vi "Main.vi"() -> ()   [LabVIEW 2017]
uses:
  <userlib>/dynamixel/dynamixel.lvlib
panel:
  in  "GO":bool
  out "Temp 2":cluster{"pos1":dbl, "pos2":dbl, "pos3":dbl}
  out "Temp":cluster{"pos1":dbl, "pos2":dbl, "pos3":dbl}
  in  "A <--> B":bool
  out "POS":cluster{"X":dbl, "Y":dbl, "Z":dbl}
  in  "Home":bool
  in  "P -> B":bool
  in  "P -> A":bool
  in  "P":cluster{"Px":dbl, "Py":dbl, "Pz":dbl}={"Px"=0.0, "Py"=0.0, "Pz"=287.0} {"Pz" format="%#.3f"; "Py" format="%#.3f"; "Px" format="%#.3f"}
  in  "A":cluster{"Bx":dbl, "By":dbl, "Bz":dbl} {"Bz" format="%#.3f"; "By" format="%#.3f"; "Bx" format="%#.3f"}
  in  "B":cluster{"Ax":dbl, "Ay":dbl, "Az":dbl} {"Az" format="%#.3f"; "Ay" format="%#.3f"; "Ax" format="%#.3f"}
  in  "Pt to Pt (GO)":bool
  in  "# of points(A to B)":i16=11
  in  "theta1a":dbl min=-150.0 max=150.0 format="%#.3f"
  in  "theta2a":dbl min=-150.0 max=150.0 format="%#.3f"
  in  "theta3a":dbl min=-150.0 max=150.0 format="%#.3f"
  in  "theta4a":dbl(knob) min=-140.0 max=140.0 scale=120.0..-120.0
  in  "devIndex":i32=46
  in  "STOP":bool
  in  "Mode Control":u16(ring) items=["Joint Space", "Cartesian Space", "Point to Point(Joint Space)", "Point to Point(Cartesian Space)", "Duplicate Position", "Home"]
  in  "constant":cluster{"d1":dbl, "a2":dbl, "a3":dbl}={"d1"=100.0, "a2"=67.0, "a3"=120.0}
  in  "ID":i16[](array[numeric])=[1, 2, 3, 4]
  # "¾÷±ñ¤âÁu±±¨îHMI"
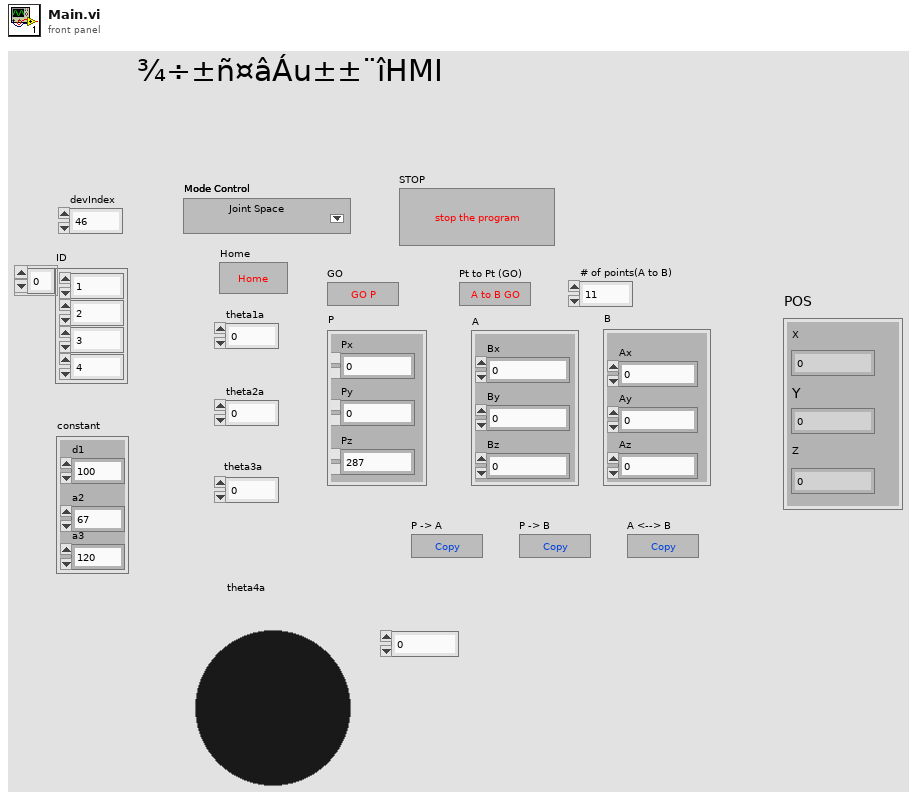
[diagram p1: front panel]
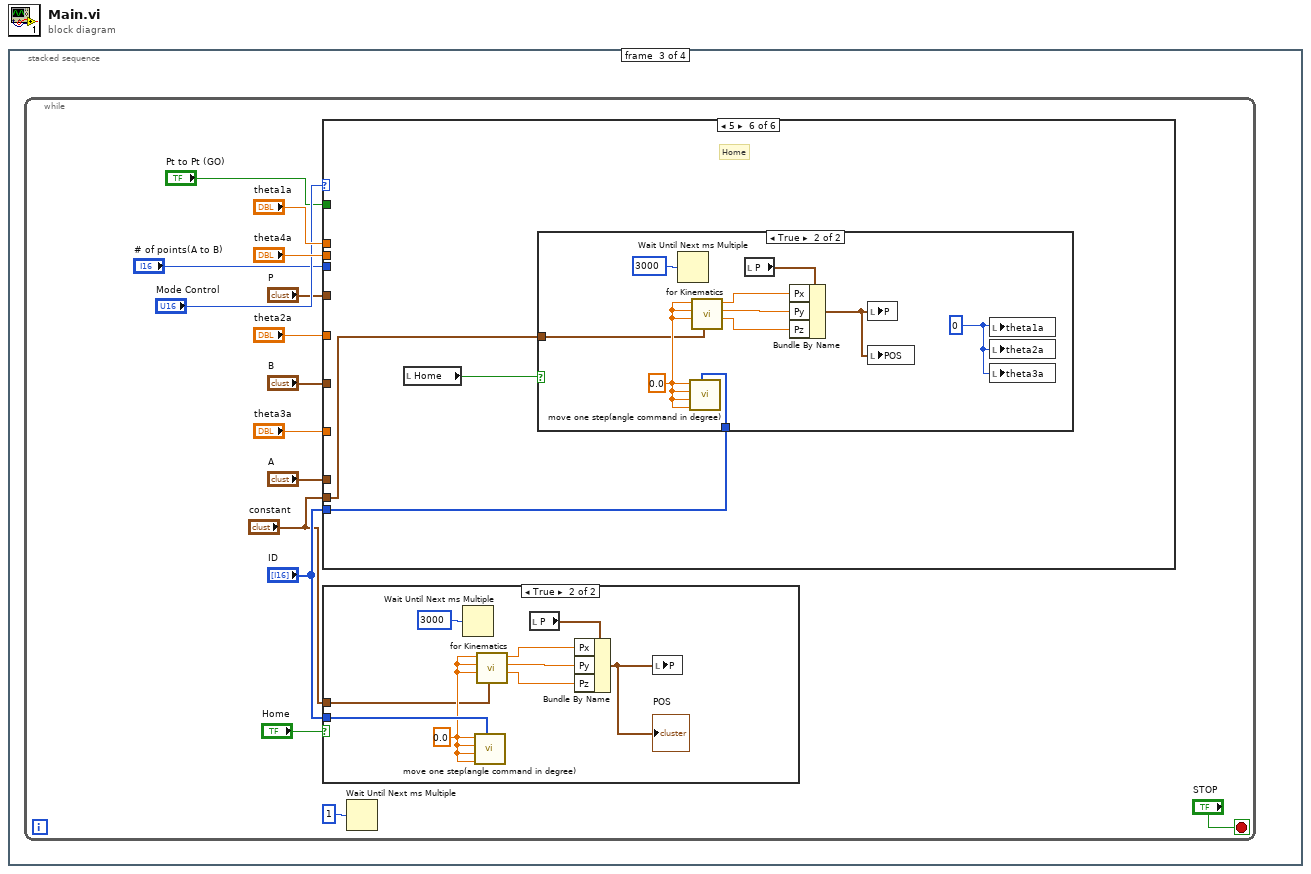
[diagram p0: block diagram]
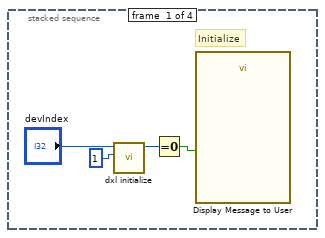
[diagram p2: hidden frame]
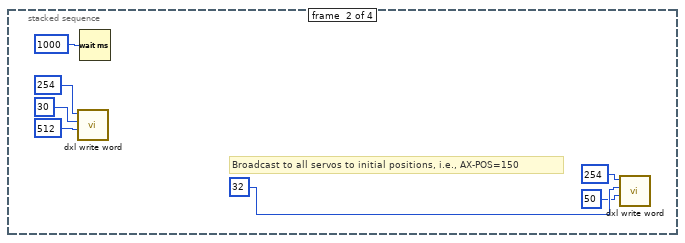
[diagram p3: hidden frame]
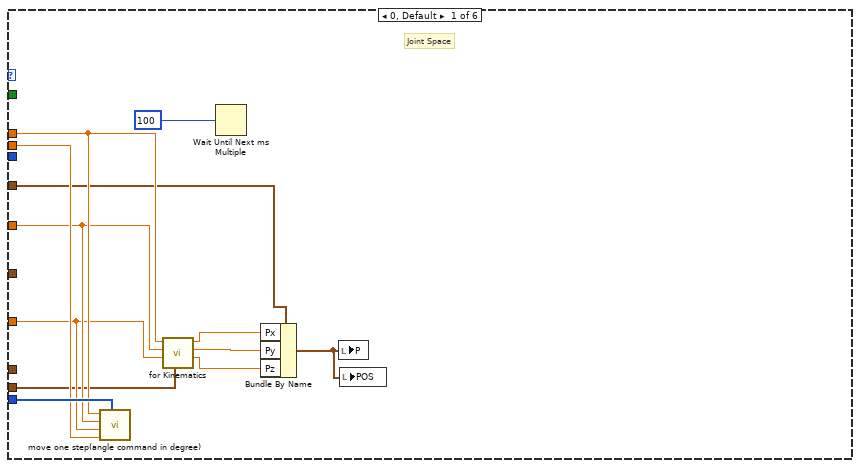
[diagram p5: hidden frame]
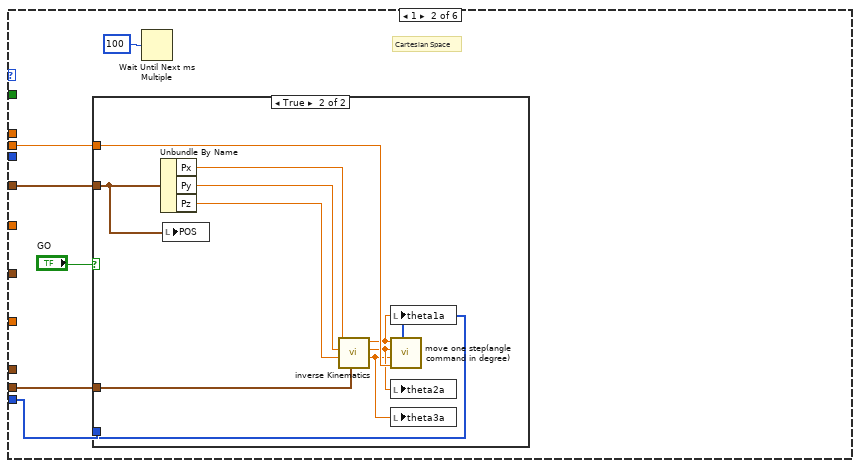
[diagram p6: hidden frame]
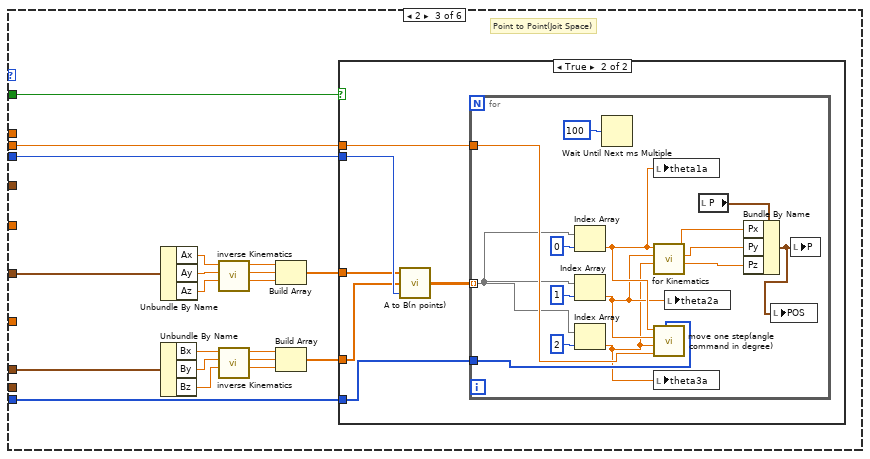
[diagram p8: hidden frame]
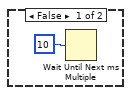
[diagram p9: hidden frame]
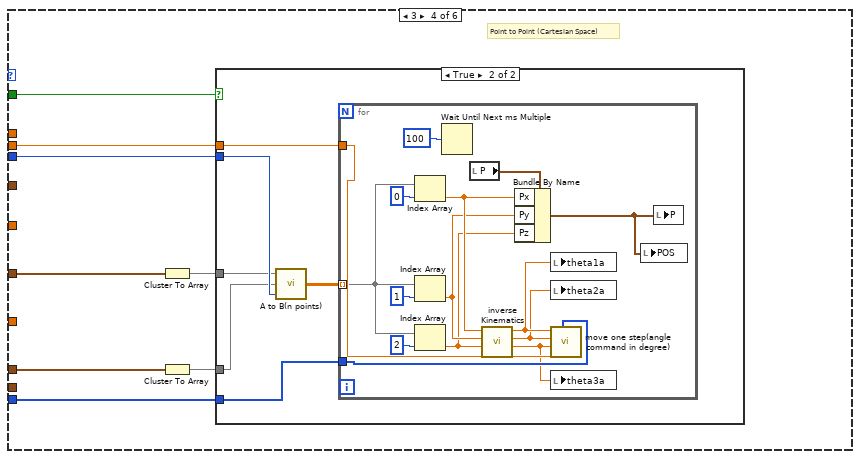
[diagram p10: hidden frame]
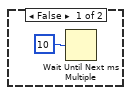
[diagram p11: hidden frame]
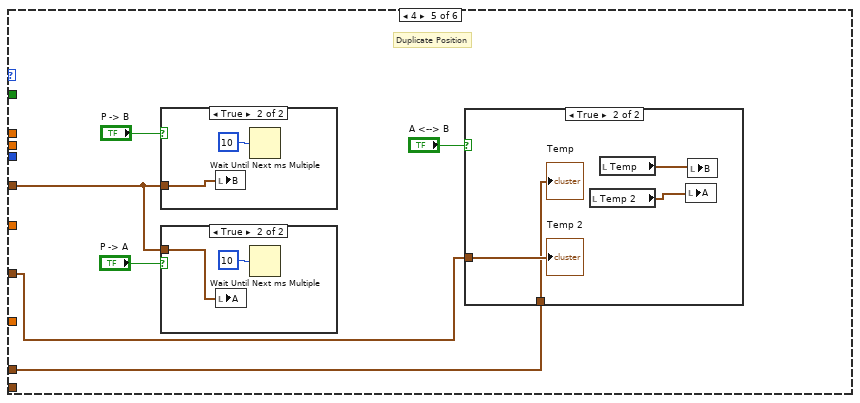
[diagram p12: hidden frame]
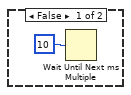
[diagram p14: hidden frame]
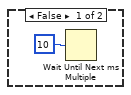
[diagram p15: hidden frame]
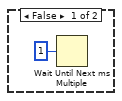
[diagram p16: hidden frame]
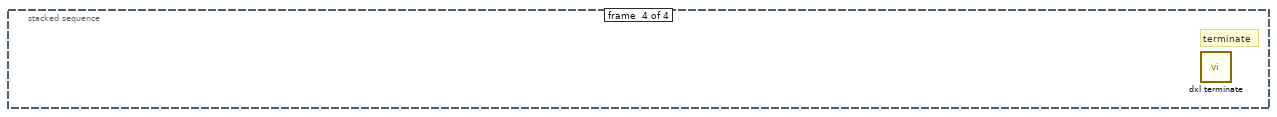
[diagram p17: hidden frame]
diagram:
  n1 = stacked-sequence {
    frame #0 {
      # "Initialize"
      n2 = call <userlib>:"dxl initialize.vi"("baudnum"=1, "devIndex"="devIndex") -> ("function return"=w3:i32)  [unwired: 9 in]
      n3 = Equal To 0?(x=w3) -> (x = 0?=w2:bool)
      n4 = call "Display Message to User"("Enable"=w2) -> ()  [unwired: 9 in, 2 out]
    }
    frame #1 {
      # "Broadcast to all servos to initial positions, i.e., AX-POS=150"
      n5 = call <userlib>:"dxl write word.vi"("value"=512, "address"=30, "id"=254) -> ()  [unwired: 9 in]
      n6 = Wait (ms)(milliseconds to wait=u32 1000) -> ()  [unwired: 1 out]
      n7 = call <userlib>:"dxl write word.vi"("value"=50, "address"=32, "id"=254) -> ()  [unwired: 9 in]
    }
    frame #2 {
      n8 = while {
        stop <- "STOP" stop-if-true
        n9 = case shown="5" "Mode Control" {
          tunnel: "theta1a" -> [w45 _ _ _ _ _]
          tunnel: "theta2a" -> [w44 _ _ _ _ _]
          tunnel: "theta3a" -> [w43 _ _ _ _ _]
          tunnel: "theta4a" -> [w46 w52 w82 w112 _ _]
          tunnel: "ID" -> [w47 w49 w83 w113 _ w153]
          tunnel: "constant" -> [w42 w53 _ _ _ w152]
          tunnel: "# of points(A to B)" -> [_ _ w81 w111 _ _]
          tunnel: "B" -> [_ _ w77 w110 w138 _]
          tunnel: "Pt to Pt (GO)" -> [_ _ w65 w107 _ _]
          tunnel: "P" -> [w37 w50 _ _ w139 _]
          tunnel: "A" -> [_ _ w64 w106 w137 _]
          frame 0, Default {
            # "Joint Space"
            n10 = call "move one step(angle command in degree).vi"("ID"=w47, "theta4a"=w46, "theta3a"=w43, "theta2a"=w44, "theta1a"=w45) -> ()  [unwired: 6 in]
            n11 = call "for Kinematics.vi"("constant"=w42, "theta3a"=w43, "theta2a"=w44, "theta1a"=w45) -> ("Pz"=w39:dbl, "Py"=w40:dbl, "Px"=w41:dbl)  [unwired: 5 in]
            n12 = Wait Until Next ms Multiple(millisecond multiple=u32 100) -> ()  [unwired: 1 out]
            n13 = Bundle By Name(cluster=w37, "Px"=w41, "Py"=w40, "Pz"=w39) -> (w36:cluster{"Px":dbl, "Py":dbl, "Pz":dbl})
            n14 = local write "P"(w36) -> ()
            n15 = local write "POS"(w36) -> ()
          }
          frame 1 {
            # "Cartesian Space"
            n16 = case shown="True" "GO" {
              tunnel: w53 -> [_ w63]
              tunnel: w52 -> [_ w62]
              tunnel: w50 -> [_ w55]
              tunnel: w49 -> [_ w54]
              frame False {
              }
              frame True {
                n17 = Unbundle By Name(w55) -> ("Px"=w58:dbl, "Py"=w57:dbl, "Pz"=w56:dbl)
                n18 = local write "POS"(w55) -> ()
                n19 = call "inverse Kinematics.vi"("constant"=w63, "Pz"=w56, "Py"=w57, "Px"=w58) -> ("theta3a"=w59:dbl, "theta2a"=w60:dbl, "theta1a"=w61:dbl)  [unwired: 5 in]
                n20 = local write "theta1a"(w61) -> ()
                n21 = call "move one step(angle command in degree).vi"("ID"=w54, "theta4a"=w62, "theta3a"=w59, "theta2a"=w60, "theta1a"=w61) -> ()  [unwired: 6 in]
                n22 = local write "theta2a"(w60) -> ()
                n23 = local write "theta3a"(w59) -> ()
              }
            }
            n24 = Wait Until Next ms Multiple(millisecond multiple=u32 100) -> ()  [unwired: 1 out]
          }
          frame 2 {
            # "Point to Point(Joit Space)"
            n25 = Unbundle By Name(w77) -> ("Ax"=w76:dbl, "Ay"=w75:dbl, "Az"=w74:dbl)
            n26 = Unbundle By Name(w64) -> ("Bx"=w80:dbl, "By"=w79:dbl, "Bz"=w78:dbl)
            n27 = call "inverse Kinematics.vi"("Pz"=w74, "Py"=w75, "Px"=w76) -> ("theta3a"=w71:dbl, "theta2a"=w72:dbl, "theta1a"=w73:dbl)  [unwired: 6 in]
            n28 = call "inverse Kinematics.vi"("Pz"=w78, "Py"=w79, "Px"=w80) -> ("theta3a"=w68:dbl, "theta2a"=w69:dbl, "theta1a"=w70:dbl)  [unwired: 6 in]
            n29 = Build Array(w73, w72, w71) -> (w66:dbl[])
            n30 = Build Array(w70, w69, w68) -> (w67:dbl[])
            n31 = case shown="True" w65 {
              tunnel: w83 -> [_ w90]
              tunnel: w82 -> [_ w89]
              tunnel: w81 -> [_ w87]
              tunnel: w67 -> [_ w85]
              tunnel: w66 -> [_ w86]
              frame False {
                n32 = Wait Until Next ms Multiple(millisecond multiple=u32 10) -> ()  [unwired: 1 out]
              }
              frame True {
                n33 = call "A to B(n points).vi"("N"=w87, "B"=w85, "A"=w86) -> ("R"=w88:dbl[][])
                n34 = for {
                  tunnel: w90 -> [w105]
                  tunnel: w89 -> [w103]
                  tunnel: w88 -> [w102] mode=indexing
                  n35 = Index Array(array=w102, index=0) -> (element=w98:dbl)
                  n36 = Index Array(array=w102, index=1) -> (element=w97:dbl)
                  n37 = Index Array(array=w102, index=2) -> (element=w96:dbl)
                  n38 = Wait Until Next ms Multiple(millisecond multiple=u32 100) -> ()  [unwired: 1 out]
                  n39 = local write "theta1a"(w98) -> ()
                  n40 = call "for Kinematics.vi"("theta3a"=w96, "theta2a"=w97, "theta1a"=w98) -> ("Pz"=w93:dbl, "Py"=w94:dbl, "Px"=w95:dbl)  [unwired: 6 in]
                  n41 = call "move one step(angle command in degree).vi"("ID"=w105, "theta4a"=w103, "theta3a"=w96, "theta2a"=w97, "theta1a"=w98) -> ()  [unwired: 6 in]
                  n42 = local write "theta3a"(w96) -> ()
                  n43 = local write "theta2a"(w97) -> ()
                  n44 = local read "P"() -> (w92:cluster{"Px":dbl, "Py":dbl, "Pz":dbl})
                  n45 = Bundle By Name(cluster=w92, "Px"=w95, "Py"=w94, "Pz"=w93) -> (w91:cluster{"Px":dbl, "Py":dbl, "Pz":dbl})
                  n46 = local write "POS"(w91) -> ()
                  n47 = local write "P"(w91) -> ()
                }
              }
            }
          }
          frame 3 {
            # "Point to Point (Cartesian Space)"
            n48 = Cluster To Array(cluster=w110) -> (array=w109:dbl[])
            n49 = Cluster To Array(cluster=w106) -> (array=w108:dbl[])
            n50 = case shown="True" w107 {
              tunnel: w113 -> [_ w120]
              tunnel: w112 -> [_ w119]
              tunnel: w111 -> [_ w117]
              tunnel: w109 -> [_ w116]
              tunnel: w108 -> [_ w115]
              frame False {
                n51 = Wait Until Next ms Multiple(millisecond multiple=u32 10) -> ()  [unwired: 1 out]
              }
              frame True {
                n52 = call "A to B(n points).vi"("N"=w117, "B"=w115, "A"=w116) -> ("R"=w118:dbl[][])
                n53 = for {
                  tunnel: w120 -> [w135]
                  tunnel: w119 -> [w133]
                  tunnel: w118 -> [w132] mode=indexing
                  n54 = Index Array(array=w132, index=0) -> (element=w125:dbl)
                  n55 = Index Array(array=w132, index=1) -> (element=w124:dbl)
                  n56 = Index Array(array=w132, index=2) -> (element=w123:dbl)
                  n57 = Wait Until Next ms Multiple(millisecond multiple=u32 100) -> ()  [unwired: 1 out]
                  n58 = local read "P"() -> (w122:cluster{"Px":dbl, "Py":dbl, "Pz":dbl})
                  n59 = call "inverse Kinematics.vi"("Pz"=w123, "Py"=w124, "Px"=w125) -> ("theta3a"=w126:dbl, "theta2a"=w127:dbl, "theta1a"=w128:dbl)  [unwired: 6 in]
                  n60 = Bundle By Name(cluster=w122, "Px"=w125, "Py"=w124, "Pz"=w123) -> (w121:cluster{"Px":dbl, "Py":dbl, "Pz":dbl})
                  n61 = local write "theta1a"(w128) -> ()
                  n62 = local write "theta2a"(w127) -> ()
                  n63 = call "move one step(angle command in degree).vi"("ID"=w135, "theta4a"=w133, "theta3a"=w126, "theta2a"=w127, "theta1a"=w128) -> ()  [unwired: 6 in]
                  n64 = local write "theta3a"(w126) -> ()
                  n65 = local write "POS"(w121) -> ()
                  n66 = local write "P"(w121) -> ()
                }
              }
            }
          }
          frame 4 {
            # "Duplicate Position"
            n67 = case shown="True" "P -> B" {
              tunnel: w139 -> [_ w147]
              frame False {
                n68 = Wait Until Next ms Multiple(millisecond multiple=u32 10) -> ()  [unwired: 1 out]
              }
              frame True {
                n69 = local write "B"(w147) -> ()
                n70 = Wait Until Next ms Multiple(millisecond multiple=u32 10) -> ()  [unwired: 1 out]
              }
            }
            n71 = case shown="True" "P -> A" {
              tunnel: w139 -> [_ w150]
              frame False {
                n72 = Wait Until Next ms Multiple(millisecond multiple=u32 10) -> ()  [unwired: 1 out]
              }
              frame True {
                n73 = local write "A"(w150) -> ()
                n74 = Wait Until Next ms Multiple(millisecond multiple=u32 10) -> ()  [unwired: 1 out]
              }
            }
            n75 = case shown="True" "A <--> B" {
              tunnel: w138 -> [_ w145]
              tunnel: w137 -> [_ w144]
              frame False {
              }
              frame True {
                n76 = local read "Temp 2"() -> (w142:cluster{"pos1":dbl, "pos2":dbl, "pos3":dbl})
                n77 = local read "Temp"() -> (w143:cluster{"pos1":dbl, "pos2":dbl, "pos3":dbl})
                n78 = local write "A"(w142) -> ()
                n79 = local write "B"(w143) -> ()
                "Temp" <- w144
                "Temp 2" <- w145
              }
            }
          }
          frame 5 {
            # "Home"
            n80 = local read "Home"() -> (w154:bool)
            n81 = case shown="True" w154 {
              tunnel: w153 -> [_ w159]
              tunnel: w152 -> [_ w158]
              frame False {
                n82 = Wait Until Next ms Multiple(millisecond multiple=u32 1) -> ()  [unwired: 1 out]
              }
              frame True {
                w156 = 0
                w165 = 0.0 ("theta1a")
                n83 = Wait Until Next ms Multiple(millisecond multiple=u32 3000) -> ()  [unwired: 1 out]
                n84 = call "move one step(angle command in degree).vi"("ID"=w159, "theta4a"=w165, "theta3a"=w165, "theta2a"=w165, "theta1a"=w165) -> ()  [unwired: 6 in]
                n85 = call "for Kinematics.vi"("constant"=w158, "theta3a"=w165, "theta2a"=w165, "theta1a"=w165) -> ("Pz"=w162:dbl, "Py"=w163:dbl, "Px"=w164:dbl)  [unwired: 5 in]
                n86 = local read "P"() -> (w160:cluster{"Px":dbl, "Py":dbl, "Pz":dbl})
                n87 = Bundle By Name(cluster=w160, "Px"=w164, "Py"=w163, "Pz"=w162) -> (w157:cluster{"Px":dbl, "Py":dbl, "Pz":dbl})
                n88 = local write "P"(w157) -> ()
                n89 = local write "POS"(w157) -> ()
                n90 = local write "theta1a"(w156) -> ()
                n91 = local write "theta2a"(w156) -> ()
                n92 = local write "theta3a"(w156) -> ()
              }
            }
          }
        }
        n93 = case shown="True" "Home" {
          tunnel: "ID" -> [_ w35]
          tunnel: "constant" -> [_ w32]
          frame False {
          }
          frame True {
            w34 = 0.0 ("theta1a")
            n94 = Wait Until Next ms Multiple(millisecond multiple=u32 3000) -> ()  [unwired: 1 out]
            n95 = call "move one step(angle command in degree).vi"("ID"=w35, "theta4a"=w34, "theta3a"=w34, "theta2a"=w34, "theta1a"=w34) -> ()  [unwired: 6 in]
            n96 = call "for Kinematics.vi"("constant"=w32, "theta3a"=w34, "theta2a"=w34, "theta1a"=w34) -> ("Pz"=w30:dbl, "Py"=w31:dbl, "Px"=w33:dbl)  [unwired: 5 in]
            n97 = local read "P"() -> (w28:cluster{"Px":dbl, "Py":dbl, "Pz":dbl})
            n98 = Bundle By Name(cluster=w28, "Px"=w33, "Py"=w31, "Pz"=w30) -> (w27:cluster{"Px":dbl, "Py":dbl, "Pz":dbl})
            "POS" <- w27
            n99 = local write "P"(w27) -> ()
          }
        }
        n100 = Wait Until Next ms Multiple(millisecond multiple=u32 1) -> ()  [unwired: 1 out]
      }
    }
    frame #3 {
      # "terminate"
      n101 = call <userlib>:"dxl terminate.vi"() -> ()  [unwired: 12 in]
    }
  }
